vi "UpdateIntTimeOnChange.vi"(8 "error in":errorcluster, 10 "Integration time [ms]":dbl(slide)=3.0 min=2.8 max=714.0 step=2.8 scale=2.8..714.0, 11 "VISA resource name in":refnum<visa-resource-name>) -> (0 "error out":errorcluster, 3 "VISA resource name out":refnum<visa-resource-name>)   [LabVIEW 2011]
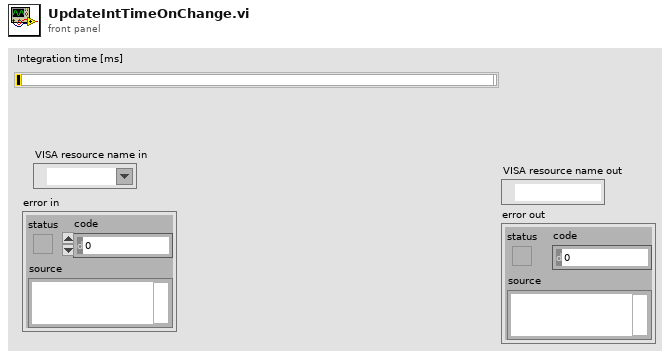
[diagram p1: front panel]
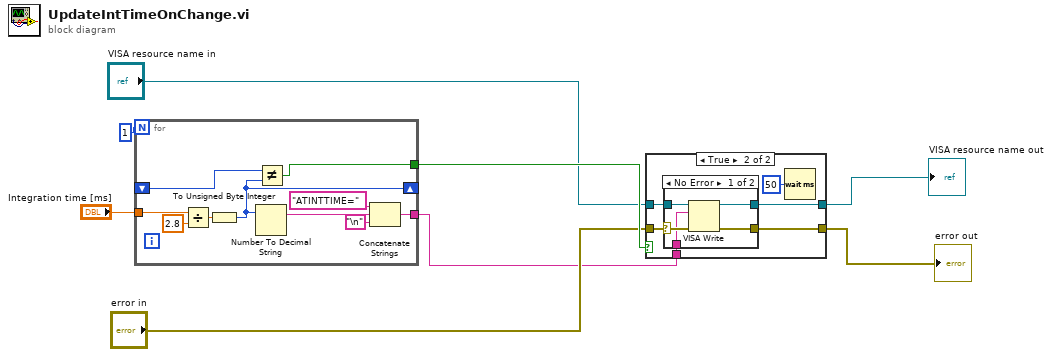
[diagram p0: block diagram]
diagram:
  n1 = for {
    N: 1 -> [_]
    shift-right: [w11] -> _
    shift-left: _ -> [w12]
    tunnel: [w9] -> w6
    tunnel: [w13] -> w1
    tunnel: "Integration time [ms]" -> [w10]
    n2 = Divide(x=w10, y=2.8) -> (x/y=w14:dbl)
    n3 = To Unsigned Byte Integer(number=w14) -> (unsigned 8bit integer=w11:u8)
    n4 = Number To Decimal String(number=w11) -> (decimal integer string=w18:string)  [unwired: 1 in]
    n5 = Not Equal?(x=w12, y=w11) -> (x != y?=w9:bool)
    n6 = Concatenate Strings("ATINTTIME=", w18, "\n") -> (w13:string)
  }
  n7 = case shown="True" w6 {
    tunnel: [w20 w26] -> w5
    tunnel: [w19 w25] -> w4
    tunnel: "VISA resource name in" -> [w20 w24]
    tunnel: "error in" -> [w19 w23]
    tunnel: w1 -> [_ w22]
    frame False {
    }
    frame True {
      n8 = case shown="No Error" w23 {
        selector: w23 -> [w28 w33]
        tunnel: [w31 w32] -> w26
        tunnel: [w30 w33] -> w25
        tunnel: w24 -> [w29 w32]
        tunnel: w22 -> [w27 _]
        frame No Error {
          n9 = VISA Write(VISA resource name=w29, write buffer=w27, error in (no error)=w28) -> (VISA resource name out=w31:refnum<visa-resource-name>, error out=w30:errorcluster)  [unwired: 1 out]
        }
        frame Error {
        }
      }
      n10 = Wait (ms)(milliseconds to wait=u32 50) -> ()  [unwired: 1 out]
    }
  }
  "VISA resource name out" <- w5
  "error out" <- w4
